vi "FindOpenAndCloseChars.vi"(8 "error in":errorcluster, 11 "String":string="TestCase {") -> (0 "error out":errorcluster, 1 "CloseChars":i32, 2 "OpenChars":i32, 3 "Counter":i32)   [LabVIEW 2013, in "CS.lvclass"]
uses:
  CS.lvclass
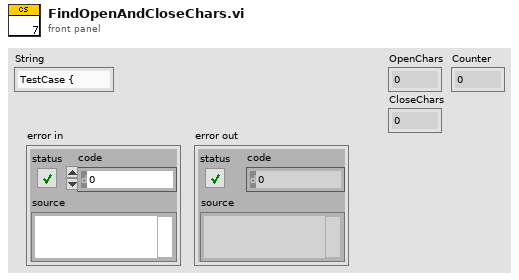
[diagram p1: front panel]
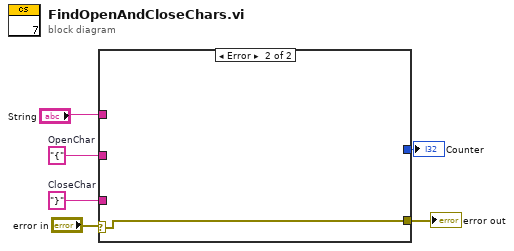
[diagram p0: block diagram]
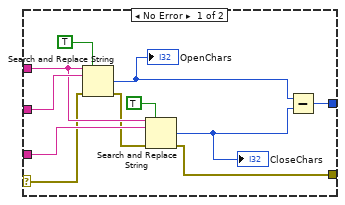
[diagram p2: hidden frame]
diagram:
  w4 = "}"  # CloseChar
  w6 = "{"  # OpenChar
  n1 = case shown="Error" "error in" {
    selector: "error in" -> [w8 w18]
    tunnel: w6 -> [w17 _]
    tunnel: "String" -> [w15 _]
    tunnel: w4 -> [w14 _]
    tunnel: [w10 _] -> w3
    tunnel: [w7 w18] -> w1
    frame No Error {
      n2 = Search and Replace String(replace all?=TRUE ("replace all? (F)"), input string=w15, search string=w17, error in=w8) -> (number of replacements=w12:i32, error out=w9:errorcluster)  [unwired: 4 in, 2 out]
      "OpenChars" <- w12
      n3 = Search and Replace String(replace all?=TRUE ("ignore case? (F)"), input string=w15, search string=w14, error in=w9) -> (number of replacements=w11:i32, error out=w7:errorcluster)  [unwired: 4 in, 2 out]
      "CloseChars" <- w11
      n4 = Subtract(x=w12, y=w11) -> (x-y=w10:i32)
    }
    frame Error {
    }
  }
  "Counter" <- w3
  "error out" <- w1
